vi "wait_to_finish_uploading.vi"(8 "error in":errorcluster, 11 "Multipart Upload in":refnum<class "Multipart Upload.lvclass">) -> (0 "error out":errorcluster, 3 "Multipart Upload out":refnum<class "Multipart Upload.lvclass">)   [LabVIEW 2020, in "Multipart Upload.lvclass"]
uses:
  Multipart Upload.lvclass
  Multipart Upload.lvclass/Multipart Upload.ctl
  Nominal Client/Nominal Client.lvclass
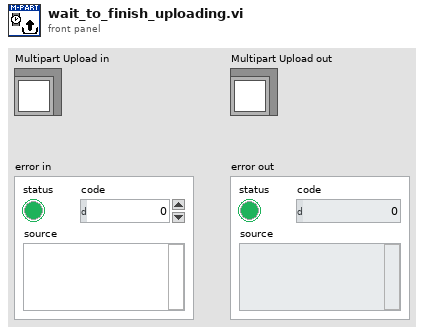
[diagram p1: front panel]
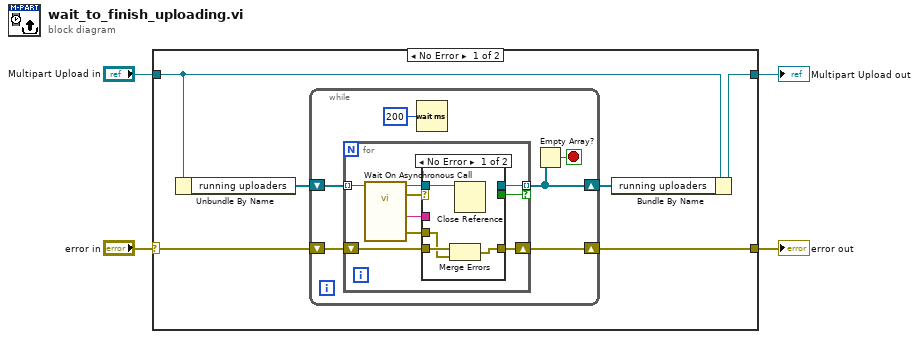
[diagram p0: block diagram]
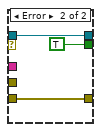
[diagram p2: hidden frame]
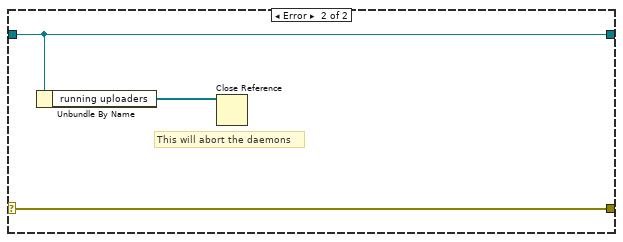
[diagram p3: hidden frame]
diagram:
  n1 = case shown="No Error" "error in" {
    selector: "error in" -> [w9 w35]
    tunnel: [w8 w35] -> w3
    tunnel: "Multipart Upload in" -> [w7 w34]
    tunnel: [w5 w34] -> w1
    frame No Error {
      n2 = Unbundle By Name(w7) -> ("running uploaders"=w10:refnum<vi>[])
      n3 = while {
        shift-right: [w11] -> w6
        shift-left: w10 -> [w16]
        shift-right: [w13] -> w8
        shift-left: w9 -> [w14]
        stop <- w15 stop-if-true
        n4 = for {
          tunnel: w16 -> [w25] mode=indexing
          tunnel: [w22] -> w11 mode=indexing if=w21
          shift-right: [w18] -> w13
          shift-left: w14 -> [w19]
          n5 = call-by-ref "Wait On Asynchronous Call"(reference=w25) -> (reference out=w23:refnum<vi>, error out=w24:errorcluster, 0:"error out"=w20:errorcluster, "Response"=w17:string)  [unwired: 11 in]
          n6 = case shown="No Error" w24 {
            tunnel: w23 -> [w29 w32]
            tunnel: [_ w32] -> w22
            tunnel: [_ TRUE] -> w21
            tunnel: w20 -> [w27 _]
            tunnel: w19 -> [w28 w30]
            tunnel: [w26 w30] -> w18
            tunnel: w17 -> [_ _]
            frame No Error {
              n7 = Merge Errors(w28, w27) -> (w26:errorcluster)
              n8 = Close Reference(reference=w29) -> ()  [unwired: 1 in, 1 out]
            }
            frame Error {
            }
          }
        }
        n9 = Wait (ms)(milliseconds to wait=u32 200) -> ()  [unwired: 1 out]
        n10 = Empty Array?(array=w11) -> (empty?=w15:bool)
      }
      n11 = Bundle By Name(cluster=w7, "running uploaders"=w6) -> (w5:refnum<class "Multipart Upload.lvclass">)
    }
    frame Error {
      # "This will abort the daemons"
      n12 = Unbundle By Name(w34) -> ("running uploaders"=w33:refnum<vi>[])
      n13 = Close Reference(reference=w33) -> ()  [unwired: 1 in, 1 out]
    }
  }
  "Multipart Upload out" <- w1
  "error out" <- w3
